vi "DSF.Engine.Execution.Builder.Command.Receive.vi"(8 "error in (no error)":errorcluster, 9 "timeout in ms (0)":i32, 11 "Builder in":refnum<class "DSF.Engine.Execution.Builder.lvclass">) -> (0 "error out":errorcluster, 1 "timed out?":bool, 2 "Command":T1={"Command"=enum."Build", "Plugin ID"=0, "Transfer ID"=0}, 3 "Builder out":refnum<class "DSF.Engine.Execution.Builder.lvclass">)   [LabVIEW 2016, in "DSF.Engine.lvlib" / "DSF.Engine.Execution.Builder.lvclass"]
uses:
  Builder/DSF.Engine.Execution.Builder.lvclass
  DSF.Engine.Execution.Builder.Command Payload.ctl
  DSF.Engine.Execution.Builder.Commands.ctl
  Builder/DSF.Engine.Execution.Builder.lvclass/DSF.Engine.Execution.Builder.ctl
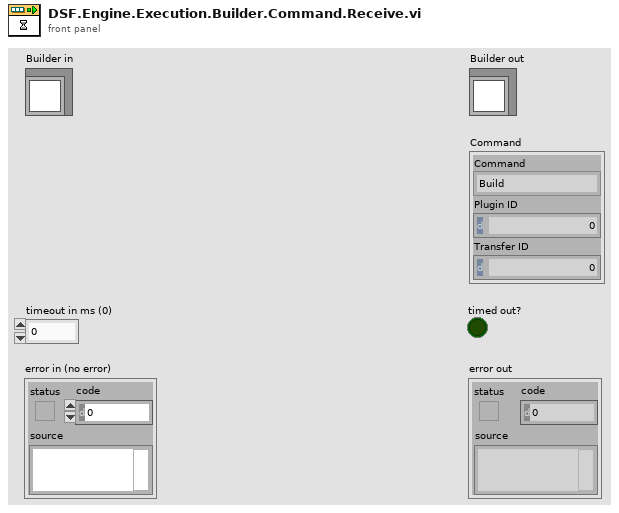
[diagram p1: front panel]
types:
  T1 = typedef "DSF.Engine.lvlib/DSF.Engine.Execution.Builder.lvclass/DSF.Engine.Execution.Builder.Command Payload.ctl" = cluster{"Command":T2, "Plugin ID":i32, "Transfer ID":i32}
  T2 = typedef "DSF.Engine.lvlib/DSF.Engine.Execution.Builder.lvclass/DSF.Engine.Execution.Builder.Commands.ctl" = enum8{"Initialize", "Build", "Parse", "Shutdown"}
  T3 = typedef "DSF.Engine.lvlib/DSF.Engine.Execution.Builder.lvclass/DSF.Engine.Execution.Builder.FIFOs.ctl" = cluster{"Command FIFO":T4, "Response FIFO":T5}
  T4 = typedef "DSF.Engine.lvlib/DSF.Engine.Execution.Builder.lvclass/DSF.Engine.Execution.Builder.Command FIFO.ctl" = refnum<k33>
  T5 = typedef "DSF.Engine.lvlib/DSF.Engine.Execution.Builder.lvclass/DSF.Engine.Execution.Builder.Response FIFO.ctl" = refnum<k33>
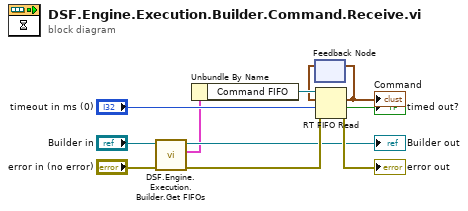
[diagram p0: block diagram]
diagram:
  n1 = call "DSF.Engine.Execution.Builder.Get FIFOs.vi"("error in (no error)"="error in (no error)", "Builder in"="Builder in") -> ("error out"=w8:errorcluster, "FIFOs"=w3:T3, "Builder out"=→"Builder out":refnum<class "DSF.Engine.Execution.Builder.lvclass">)  [unwired: 7 in]
  n2 = Unbundle By Name(w3) -> ("Command FIFO"=w9:T4)
  n3 = feedback #1() -> (w1:T1)  [unwired: 1 in]
  n4 = RT FIFO Read(0:w9, 1:w1, 2:"timeout in ms (0)", 3:w8) -> (9:w2:T1, 10:→"timed out?":bool, 11:→"error out":errorcluster)  [unwired: 2 out]
  "Command" <- w2
  n5 = feedback-in #1(w2) -> ()
